vi "test Action Update Ramp Rate-RampRate30.vi"() -> ()   [LabVIEW 2018, in "AllComponentTestes.lvclass"]
uses:
  AllComponentTestes.lvclass
  C:/Program Files/National Instruments/LabVIEW 2018/vi.lib/addons/_JKI Toolkits/VI Tester/TestCase.llb/TestCase.lvclass
  <vilib>/addons/_JKI Toolkits/VI Tester/TestCase.llb/TestCase.lvclass
  Libraries/Thermal Chamber Controller_DQMH/Thermal Chamber Controller_DQMH.lvlib
panel:
  out "TestCase out":refnum<class "TestCase.lvclass">
  in  "TestCase in":refnum<class "AllComponentTestes.lvclass">
  out "error out":errorcluster
  in  "error in (no error)":errorcluster
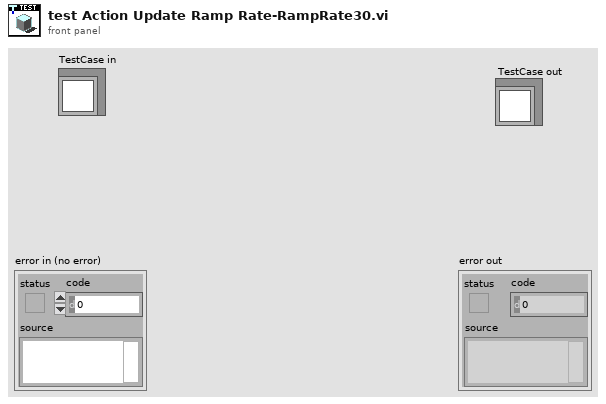
[diagram p1: front panel]
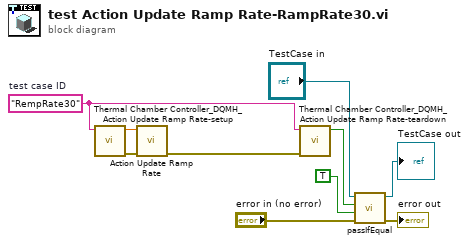
[diagram p0: block diagram]
diagram:
  w5 = "RempRate30"  # test case ID
  n1 = call "Thermal Chamber Controller_DQMH_Action Update Ramp Rate-setup.vi"("test case ID"=w5) -> ("error in"=w7:errorcluster, "Temperature Ramp Rate"=w8:dbl)  [unwired: 9 in]
  n2 = call "Action Update Ramp Rate.vi"("error in (no error)"=w7, "Temperature Ramp Rate"=w8) -> ("error out"=w6:errorcluster)  [unwired: 9 in]
  n3 = call "Thermal Chamber Controller_DQMH_Action Update Ramp Rate-teardown.vi"("error out"=w6, "test case ID"=w5) -> ("result"=w4:bool)  [unwired: 9 in]
  n4 = call-dynamic "passIfEqual.vi"("error in (no error)"="error in (no error)", "y"=TRUE, "x"=w4, "TestCase in"="TestCase in") -> ("error out"=→"error out":errorcluster, "TestCase out"=→"TestCase out":refnum<class "AllComponentTestes.lvclass">)  [unwired: 6 in]
